vi "opctank.vi"(1 "h":dbl, 2 "connection in":string) -> (0 "connection out":string)   [LabVIEW 2021]
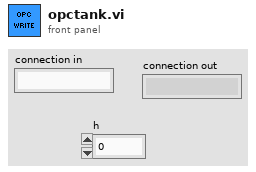
[diagram p1: front panel]
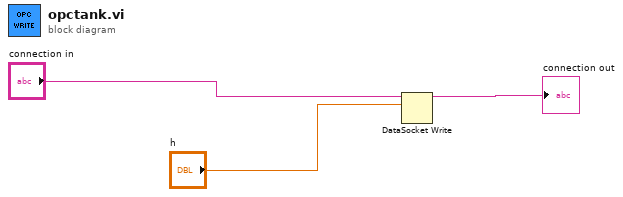
[diagram p0: block diagram]
diagram:
  n1 = DataSocket Write(10:"h", 11:"connection in") -> (3:→"connection out":string)  [unwired: 2 in, 2 out]
